vi "Enqueue Direction.vi"(6 "Index in":i64, 9 "Velocity in":dbl, 10 "Direction in":cluster{dbl, dbl}, 11 "Communication in":refnum<class "Communication.lvclass">) -> ()   [LabVIEW 2024, in "Communication.lvclass"]
doc: "MIT Licence\nCopyright (c) 2024 David Grollier"
uses:
  Communication.lvclass
  Communication.lvclass/Communication.ctl
  Game Componants/Game Board/State Command.ctl
  Game Componants/Game Board/Game Board.lvclass
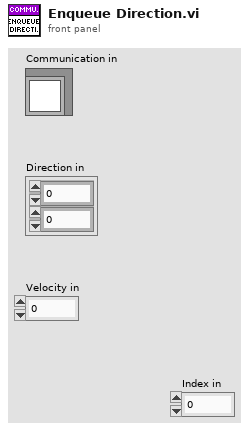
[diagram p1: front panel]
types:
  T1 = typedef "Game Board.lvclass/State Command.ctl" = cluster{"Direction":cluster{dbl, dbl}, "Velocity":dbl}
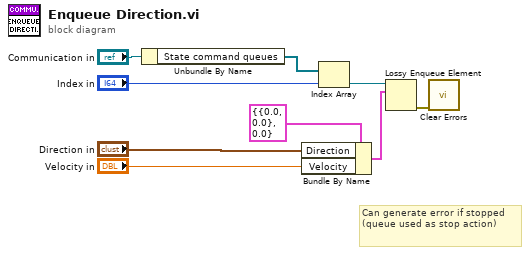
[diagram p0: block diagram]
diagram:
  # "Can generate error if stopped (queue used as stop action)"
  n1 = Unbundle By Name("Communication in") -> ("State command queues"=w8:refnum<queue>[])
  n2 = Bundle By Name(cluster=T1 {"Direction"={0.0, 0.0}, "Velocity"=0.0} ("element"), "Direction"="Direction in", "Velocity"="Velocity in") -> (w2:T1)
  n3 = Index Array(array=w8, index="Index in") -> (element=w6:refnum<queue>)
  n4 = Lossy Enqueue Element(queue=w6, element=w2) -> (error out=w1:errorcluster)  [unwired: 1 in, 3 out]
  n5 = call <vilib>:"Clear Errors.vi"("error in (no error)"=w1) -> ()  [unwired: 5 in, 2 out]
